vi "Generic Datatype to NI DataType.vi"(11 "Generic Datatype":T2=enum."Bool") -> (3 "NI Datatype":T1)   [LabVIEW 2021, in "DataTypes_CIF_U.lvlib"]
doc: "Convert generic datatypes into NI datatypes."
uses:
  DataTypes_CIF_U.lvlib
  <vilib>/Utility/Data Type/Type Definitions/Data Type.ctl
  <vilib>/Utility/Data Type/NI_Data Type.lvlib
  Typedef/Generic Datatypes.ctl
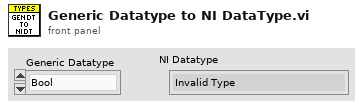
[diagram p1: front panel]
types:
  T1 = typedef "NI_Data Type.lvlib/Data Type.ctl" = enum8{"Invalid Type", "Void", "I8", "I16", "I32", "I64", "U8", "U16", "U32", "U64", "Single Float", "Double Float", "Extended Float", "Single Complex", "Double Complex", "Extended Complex", "Enum U8", "Enum U16", "Enum U32", "Enum U64", "Single Float With Unit", "Double Float With Unit", "Extended Float With Unit", "Single Complex with Unit", "Double Complex with Unit", "Extended Complex with Unit", "Boolean", "String", "Path", "Picture", "Tag", "Array", "Cluster", "Variant", "LV Variant", "Waveform", "Timestamp", "Digital Waveform", "Digital Data", "ExpressData", "Refnum", "External Data", "VI", "Poly VI", "LabVIEW Class Instance", "Fixed Point", "Set Collection", "Map Collection"}
  T2 = typedef "DataTypes_CIF_U.lvlib/Generic Datatypes.ctl" = enum16{"Invalid", "Bool", "U8", "I8", "U16", "I16", "U32", "I32", "U64", "I64", "Single Float", "Double Float", "String"}
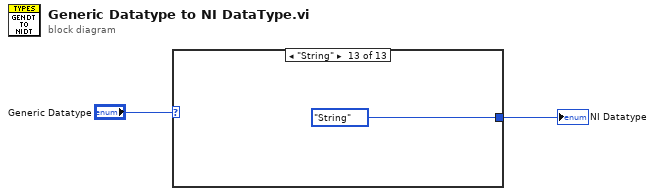
[diagram p0: block diagram]
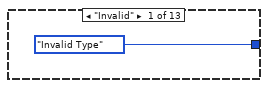
[diagram p2: hidden frame]
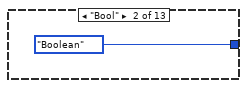
[diagram p3: hidden frame]
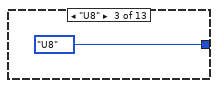
[diagram p4: hidden frame]
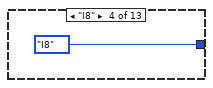
[diagram p5: hidden frame]
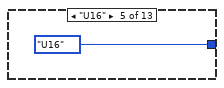
[diagram p6: hidden frame]
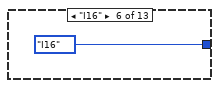
[diagram p7: hidden frame]
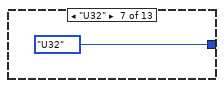
[diagram p8: hidden frame]
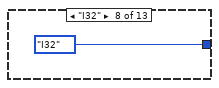
[diagram p9: hidden frame]
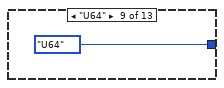
[diagram p10: hidden frame]
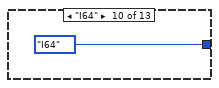
[diagram p11: hidden frame]
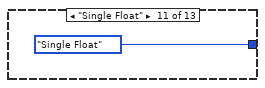
[diagram p12: hidden frame]
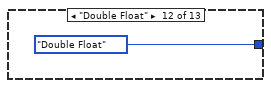
[diagram p13: hidden frame]
diagram:
  n1 = case shown="\"String\"" "Generic Datatype" {
    tunnel: [Data_Type."Invalid Type" ("NI Datatype") Data_Type."Boolean" ("NI Datatype") Data_Type."U8" ("NI Datatype") Data_Type."I8" ("NI Datatype") Data_Type."U16" ("NI Datatype") Data_Type."I16" ("NI Datatype") Data_Type."U32" ("NI Datatype") Data_Type."I32" ("NI Datatype") Data_Type."U64" ("NI Datatype") Data_Type."I64" ("NI Datatype") Data_Type."Single Float" ("NI Datatype") Data_Type."Double Float" ("NI Datatype") Data_Type."String" ("NI Datatype")] -> w1
    frame "Invalid" {
    }
    frame "Bool" {
    }
    frame "U8" {
    }
    frame "I8" {
    }
    frame "U16" {
    }
    frame "I16" {
    }
    frame "U32" {
    }
    frame "I32" {
    }
    frame "U64" {
    }
    frame "I64" {
    }
    frame "Single Float" {
    }
    frame "Double Float" {
    }
    frame "String" {
    }
  }
  "NI Datatype" <- w1
